vi "Keithley 6517 Initialize.vi"(2 "error in (no error)":errorcluster, 3 "GPIB Address":string="27") -> (0 "error out copy":errorcluster, 1 "Instrument ID String":string="KEITHLEY INSTRUMENTS INC.,MODEL 6517B,1253950,A06/700x \n")   [LabVIEW 2024]
doc: "This VI Sets the parameters of the GPIB Interface for Re-Addressing, Assert REN and System controller. You must run this VI before using any of the instrument driver VIs for this instrument."
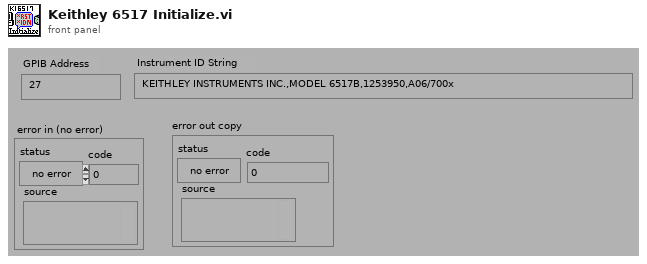
[diagram p1: front panel]
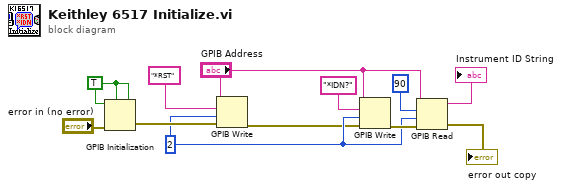
[diagram p0: block diagram]
diagram:
  w6 = 2
  w12 = TRUE
  n1 = GPIB Initialization(1:w12, 3:w12, 4:"error in (no error)", 7:w12) -> (0:w11:errorcluster)  [unwired: 3 in]
  n2 = GPIB Write(0:"GPIB Address", 1:"*RST", 2:w6, 3:w11) -> (6:w1:errorcluster)  [unwired: 1 in, 1 out]
  n3 = GPIB Write(0:"GPIB Address", 1:"*IDN?", 2:w6, 3:w1) -> (6:w7:errorcluster)  [unwired: 1 in, 1 out]
  n4 = GPIB Read(0:"GPIB Address", 1:90, 2:w6, 3:w7) -> (5:→"Instrument ID String":string, 7:→"error out copy":errorcluster)  [unwired: 1 in, 1 out]
